vi "MIMO Calculation.vi"(2 "x(n)":dbl[](array[numeric]) format="%.2f", 3 "MIMO State-Space":T1 {"D" format="%.2f"; "C" format="%.2f"; "B" format="%.2f"; "A" format="%.2f"}, 4 "u(n)":dbl[](array[numeric]) format="%.2f") -> (0 "y(n)":dbl[](array[numeric]) format="%.2f", 1 "x(n+1)":dbl[](array[numeric]) format="%.2f")   [LabVIEW 2017, in "NI_AdvCtrl_continuous linear.lvlib"]
doc: "LabVIEW no longer supports this VI. You can obtain similar functionality by installing the LabVIEW Simulation Module."
uses:
  <vilib>/addons/control/advanced/NI_AdvCtrl_continuous linear.lvlib
  <vilib>/Analysis/baseanly.llb/A x Vector.vi
  <vilib>/Analysis/NI_AALBase.lvlib
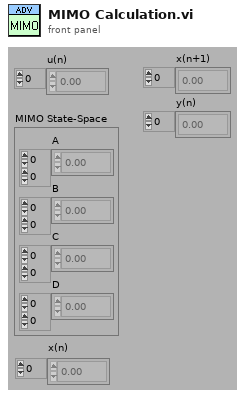
[diagram p1: front panel]
types:
  T1 = cluster{"A":dbl[][], "B":dbl[][], "C":dbl[][], "D":dbl[][]}
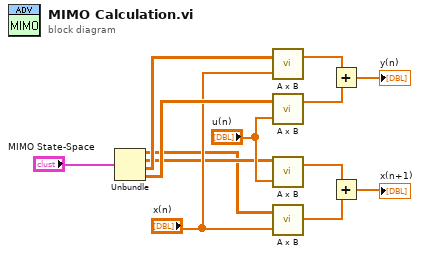
[diagram p0: block diagram]
diagram:
  n1 = Unbundle("MIMO State-Space") -> ("A"=w4:dbl[][], "B"=w5:dbl[][], "C"=w9:dbl[][], "D"=w11:dbl[][])
  n2 = call-poly <vilib>:"A x B.vi"("Vector"="x(n)", "A"=w9) -> ("A x Vector"=w13:dbl[])  [unwired: 1 out]
  n3 = call-poly <vilib>:"A x B.vi"("Vector"="u(n)", "A"=w11) -> ("A x Vector"=w8:dbl[])  [unwired: 1 out]
  n4 = call-poly <vilib>:"A x B.vi"("Vector"="u(n)", "A"=w5) -> ("A x Vector"=w6:dbl[])  [unwired: 1 out]
  n5 = call-poly <vilib>:"A x B.vi"("Vector"="x(n)", "A"=w4) -> ("A x Vector"=w7:dbl[])  [unwired: 1 out]
  n6 = Add(x=w13, y=w8) -> (x+y=→"y(n)":dbl[])
  n7 = Add(x=w6, y=w7) -> (x+y=→"x(n+1)":dbl[])
